vi "Rotate_Angle.vi"(7 "Direction of Rotation":T1, 8 "error in (no error)":errorcluster, 10 "Angle.lvclass":refnum<class "Angle.lvclass">, 11 "PolarVector in":refnum<class "PolarVector.lvclass">) -> (0 "error out":errorcluster, 3 "PolarVector out":refnum<class "PolarVector.lvclass">)   [LabVIEW 2011, in "PolarVector.lvclass"]
uses:
  PolarVector.lvclass
  TypeDefs/DirectionOfRotation.ctl
  Angles/Angle/Angle.lvclass
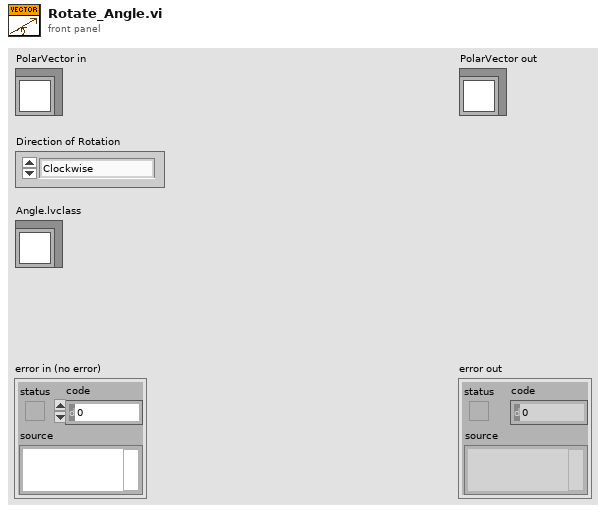
[diagram p1: front panel]
types:
  T1 = typedef "DirectionOfRotation.ctl" = enum16{"Clockwise", "Counter-Clockwise"}
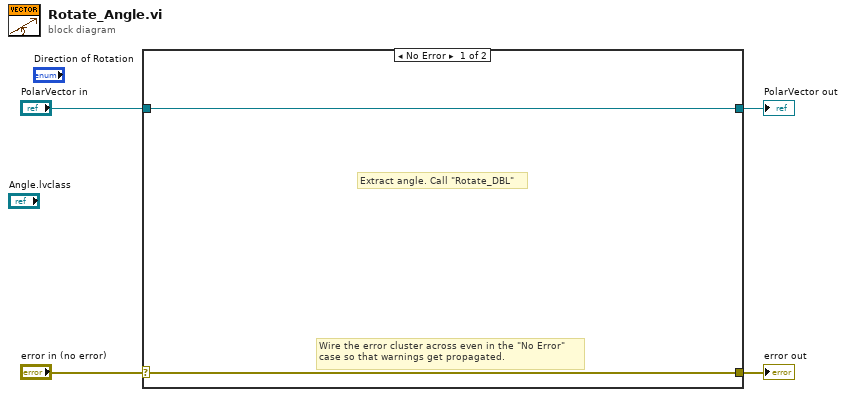
[diagram p0: block diagram]
diagram:
  n1 = case shown="No Error" "error in (no error)" {
    selector: "error in (no error)" -> [w5 w8]
    tunnel: [w5 w8] -> w3
    tunnel: [w6 w7] -> w1
    tunnel: "PolarVector in" -> [w6 w7]
    frame No Error {
      # "Extract angle. Call \"Rotate_DBL\""
      # "Wire the error cluster across even in the \"No Error\"\ncase so that warnings get propagated."
    }
    frame Error {
    }
  }
  "error out" <- w3
  "PolarVector out" <- w1
